vi "Load Config.vi"(6 "Constants":refnum<class "Sequence Constants.lvclass">, 8 "error in (no error)":refnum<class "MultiErrors.lvclass">, 10 "Config Element":refnum<class "Config Element.lvclass">, 11 "Start Log Command Config in":refnum<class "Start Log Command Config.lvclass">) -> (0 "error out":refnum<class "MultiErrors.lvclass">, 3 "Start Log Command Config out":refnum<class "Start Log Command Config.lvclass">)   [LabVIEW 2020, in "VolatusSeqConfig.lvlib" / "Start Log Command Config.lvclass"]
uses:
  Start Log Command Config.lvclass
  VolatusErrorUtilities/MultiErrors/MultiErrors.lvclass
  lv-cdm/CDM-Config/Config Element/Config Element.lvclass
  Start Log Command Config.lvclass/Start Log Command Config.ctl
  Sequence Constants/Sequence Constants.lvclass
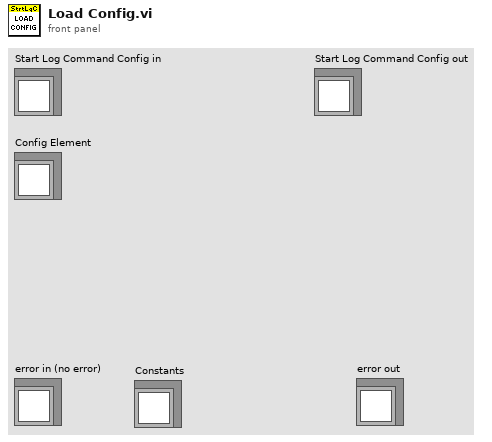
[diagram p1: front panel]
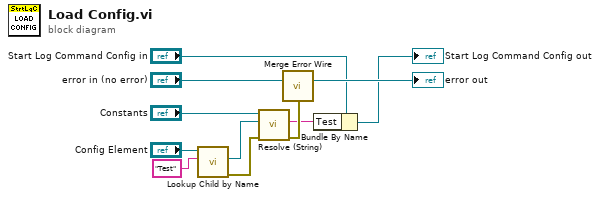
[diagram p0: block diagram]
diagram:
  n1 = call "Lookup Child by Name.vi"("Name"="Test", "Config Element in"="Config Element") -> ("error out"=w2:errorcluster, "Child"=w3:refnum<class "Config Element.lvclass">)  [unwired: 6 in, 2 out]
  n2 = call "Resolve (String).vi"("error in (no error)"=w2, "Element"=w3, "Sequence Constants in"="Constants") -> ("error out"=w11:errorcluster, "String Value"=w1:string)  [unwired: 6 in, 1 out]
  n3 = call "Merge Error Wire.vi"("error in (no error)"=w11, "MultiErrors in"="error in (no error)") -> ("MultiErrors out"=→"error out":refnum<class "MultiErrors.lvclass">)  [unwired: 13 in]
  n4 = Bundle By Name(cluster="Start Log Command Config in", "Test"=w1) -> (→"Start Log Command Config out":refnum<class "Start Log Command Config.lvclass">)
